vi "Get Default Name From TD.vi"(8 "错误输入":errorcluster, 10 "Type Descriptor":T1) -> (0 "错误输出":errorcluster, 2 "Name":string)   [LabVIEW 2012, in "TD Tools.lvlib"]
uses:
  TD Tools.lvlib
  Custom Type/Type Descriptor.ctl
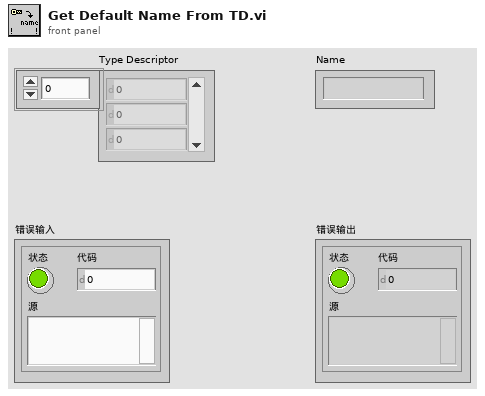
[diagram p1: front panel]
types:
  T1 = typedef "TD Tools.lvlib/Type Descriptor.ctl" = u16[]
  T2 = typedef "TD Tools.lvlib/Type Descriptor Header.ctl" = cluster{"length":u16, "private":u8, "type":T3, "# elements":u16}
  T3 = typedef "TD Tools.lvlib/Type Descriptor Enumeration.ctl" = enum16{"<Null>", "I8", "I16", "I32", "I64", "U8", "U16", "U32", "U64", "SGL", "DBL", "EXT", "CSG", "CDB", "CXT", "0x0F", "0x10", "0x11", "0x12", "0x13", "0x14", "Enum U8", "Enum U16", "Enum U32", "Enum U64", "SGL PQ", "DBL PQ", "EXT PQ", "CSG PQ", "CDB PQ", "CXT PQ", "0x1F", "0x20", "Boolean", "0x22", "0x23", "0x24", "0x25", "0x26", "0x27", "0x28", "0x29", "0x2A", "0x2B", "0x2C", "0x2D", "0x2E", "0x2F", "String", "0x31", "Path", "Pict", "0x34", "0x35", "0x36", "DAQ", "0x38", "0x39", "0x3A", "0x3B", "0x3C", "0x3D", "0x3E", "0x3F", "Array", "0x41", "0x42", "0x43", "0x44", "0x45", "0x46", "0x47", "0x48", "0x49", "0x4A", "0x4B", "0x4C", "0x4D", "0x4E", "0x4F", "Cluster", "0x51", "0x52", "Variant", "Waveform", "0x55", "0x56", "0x57", "0x58", "0x59", "0x5A", "0x5B", "0x5C", "0x5D", "0x5E", "0x5F", "0x60", "0x61", "0x62", "0x63", "0x64", "0x65", "0x66", "0x67", "0x68", "0x69", "0x6A", "0x6B", "0x6C", "0x6D", "0x6E", "0x6F", "Refnum"}
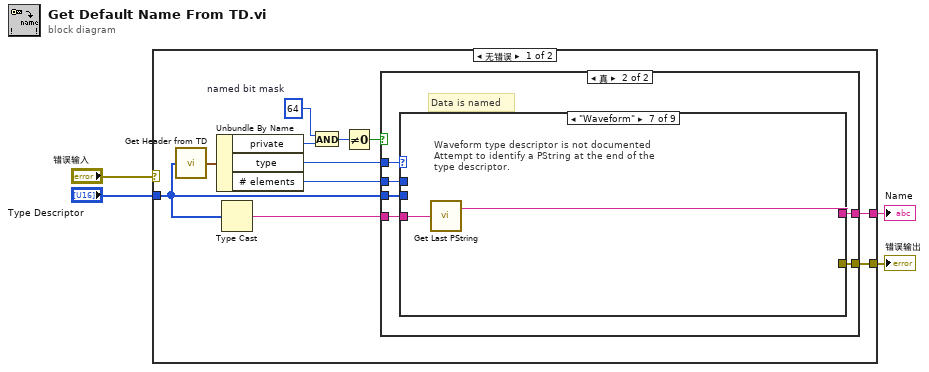
[diagram p0: block diagram]
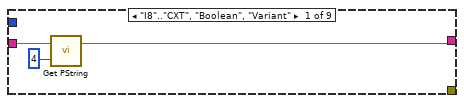
[diagram p3: hidden frame]
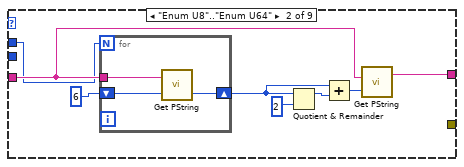
[diagram p4: hidden frame]
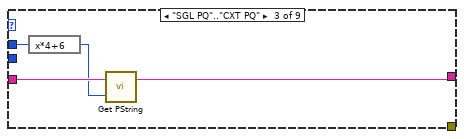
[diagram p5: hidden frame]
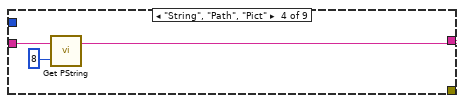
[diagram p6: hidden frame]
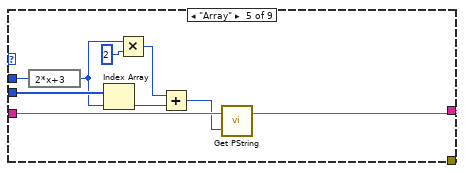
[diagram p7: hidden frame]
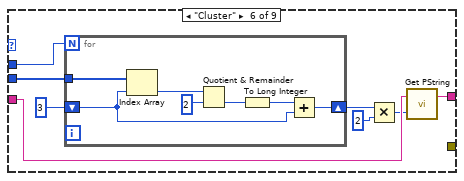
[diagram p8: hidden frame]
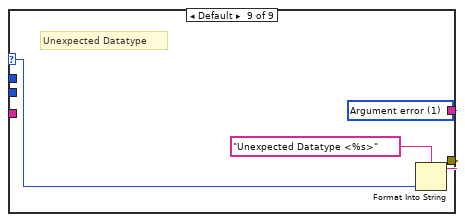
[diagram p10: hidden frame]
diagram:
  n1 = case shown="无错误" "错误输入" {
    selector: "错误输入" -> [_ w77]
    tunnel: "Type Descriptor" -> [w14 _]
    tunnel: [w11 "" ("Last PString")] -> w3
    tunnel: [w5 w77] -> w1
    frame No Error {
      w8 = u8 64  # named bit mask
      n2 = call "Get Header from TD.vi"("Type Desciptor"=w14) -> ("Type Descriptor Header"=w15:T2)
      n3 = Unbundle By Name(w15) -> ("private"=w7:u8, "type"=w6:T3, "# elements"=w13:u16)
      n4 = Type Cast(x=w14) -> (*(type *) &x=w12:string)  [unwired: 1 in]
      n5 = And(x=w8, y=w7) -> (x .and. y?=w10:u8)
      n6 = Not Equal To 0?(x=w10) -> (x != 0?=w9:bool)
      n7 = case shown="真" w9 {
        tunnel: [_ w21] -> w5
        tunnel: w6 -> [_ w20]
        tunnel: w12 -> [_ w19]
        tunnel: [_ w18] -> w11
        tunnel: w13 -> [_ w17]
        tunnel: w14 -> [_ w16]
        frame False {
        }
        frame True {
          # "Data is named"
          n8 = case shown="\"Waveform\"" w20 {
            selector: w20 -> [_ _ _ _ _ _ _ _ w71]
            tunnel: [_ _ _ _ _ _ _ _ w75] -> w21
            tunnel: w19 -> [w24 w29 w38 w42 w49 w57 w68 w70 _]
            tunnel: [w22 w28 w36 w41 w48 w56 w67 w69 _] -> w18
            tunnel: w17 -> [_ w27 w39 _ w51 w59 _ _ _]
            tunnel: w16 -> [_ _ _ _ w50 w58 _ _ _]
            frame "I8".."CXT", "Boolean", "Variant" {
              n9 = call "Get PString.vi"("offset(0)"=4 ("offset (0)"), "String"=w24) -> ("PString"=w22:string)  [unwired: 1 out]
            }
            frame "Enum U8".."Enum U64" {
              n10 = for {
                N: w27 -> [_]
                tunnel: w29 -> [w33]
                shift-right: [w34] -> w31
                shift-left: 6 -> [w35]
                n11 = call "Get PString.vi"("offset(0)"=w35, "String"=w33) -> ("offset  Past PString"=w34:i32)  [unwired: 1 out]
              }
              n12 = Quotient & Remainder(x=w31, y=2) -> (x-y*floor(x/y)=w25:i32)  [unwired: 1 out]
              n13 = Add(x=w31, y=w25) -> (x+y=w30:i32)
              n14 = call "Get PString.vi"("offset(0)"=w30, "String"=w29) -> ("PString"=w28:string)  [unwired: 1 out]
            }
            frame "SGL PQ".."CXT PQ" {
              n15 = expression code="x*4+6"(w39) -> (w37:u16)
              n16 = call "Get PString.vi"("offset(0)"=w37, "String"=w38) -> ("PString"=w36:string)  [unwired: 1 out]
            }
            frame "String", "Path", "Pict" {
              n17 = call "Get PString.vi"("offset(0)"=8 ("offset (0)"), "String"=w42) -> ("PString"=w41:string)  [unwired: 1 out]
            }
            frame "Array" {
              n18 = expression code="2*x+3"(w51) -> (w47:u16)
              n19 = Index Array(array=w50, index=w47) -> (element=w44:u16)
              n20 = Multiply(x=w47, y=u16 2) -> (x*y=w45:u16)
              n21 = Add(x=w45, y=w44) -> (x+y=w43:u16)
              n22 = call "Get PString.vi"("offset(0)"=w43, "String"=w49) -> ("PString"=w48:string)  [unwired: 1 out]
            }
            frame "Cluster" {
              n23 = for {
                N: w59 -> [_]
                shift-right: [w65] -> w54
                shift-left: 3 -> [w64]
                tunnel: w58 -> [w66]
                n24 = Index Array(array=w66, index=w64) -> (element=w62:u16)
                n25 = Quotient & Remainder(x=w62, y=i16 2) -> (floor(x/y)=w63:u16)  [unwired: 1 out]
                n26 = To Long Integer(number=w63) -> (32bit integer=w60:i32)
                n27 = Add(x=w60, y=w64) -> (x+y=w65:i32)
              }
              n28 = Multiply(x=w54, y=2) -> (x*y=w53:i32)
              n29 = call "Get PString.vi"("offset(0)"=w53, "String"=w57) -> ("PString"=w56:string)  [unwired: 1 out]
            }
            frame "Waveform" {
              # "Waveform type descriptor is not documented\nAttempt to identify a PString at the end of the\ntype descriptor."
              n30 = call "Get Last PString.vi"("String"=w68) -> ("Last String"=w67:string)  [unwired: 1 out]
            }
            frame "DAQ", "Refnum" {
              # "Refnums type descriptors are not documented\nAttempt to identify a PString at the end of the\ntype descriptor."
              n31 = call "Get Last PString.vi"("String"=w70) -> ("Last String"=w69:string)  [unwired: 1 out]
            }
            frame Default {
              w74 = 1 items=["No error", "Argument error", "Memory is full", "Out of zone", "End of file", "File already open", "Generic file I/O error", "File not found", "File permission error", "Disk is full", "Duplicate path", "Too many files open", "System feature not enabled", "Resource file not found", "Cannot add resource", "Resource not found", "Image not found", "Image memory error", "Pen does not exist", "Config type invalid", "Config token not found", "Config parse error", "Config memory error", "Bad external code format", "Bad external code offset", "External code not present", "Null window", "Destroy window error", "Null menu", "Print aborted", "Bad print record", "Print driver error", "Windows error during printing", "Memory error during printing", "Print dialog error", "Generic print error", "Invalid device refnum", "Device not found", "Device parameter error", "Device unit error", "Cannot open device", "Device call aborted", "Generic error", "Cancelled by user", "Object ID too low", "Object ID too high", "Object not in heap", "Unknown heap", "Unknown object (invalid DefProc)", "Unknown object (DefProc not in table)", "Message out of range", "Invalid (null) method", "Unknown message", "Manager call not supported", "Bad address", "Network operation in progress", "Network operation timed out", "Connection is busy", "Network attribute not supported", "Network error", "Address in use", "System out of memory", "Connection aborted", "Connection refused", "Not connected", "Already connected", "Connection closed", "Initialization error (interapplication manager)", "Bad occurrence", "Wait on unbound occurrence handler", "Occurrence queue overflow", "Datalog type conflict", "Unused", "Unrecognized type (interapplication manager)", "Memory corrupt", "Failed to make temporary DLL", "Old CIN version", "Drag socket not found", "Failed to load drop-object", "Failed to register OLE object", "Failed to release OLE object", "Format specifier type mismatch", "Unknown format specifier", "Too few format specifiers", "Too many format specifiers", "Scan failed", "Newer CIN version", "Error converting to variant", "Runtime menu error", "Password tampered", "Variant attribute not found", "Incompatible variant data type", "Event data is not available", "Event Store is not present", "Occurrence is not found", "Event Queue is not created", "Event info is not available", "Refnum passed is NULL", "Error retrieving Class GUID", "Error retrieving CoClass GUID", "Error retrieving TypeLib GUID.", "Bad built application magic bytes.", "Specific driver is different from the specific driver associated with the Logical Name.", "There is no session opened to the class driver.", "Max Error", "MAX - Error with config objects", "MAX - Error loading configuration", "MAX - Group not supported"]
              # "Unexpected Datatype"
              n32 = Format Into String(format string="Unexpected Datatype <%s>" ("Format String"), w71) -> (resulting string=w72:string)  [unwired: 2 in, 1 out]
              n33 = call "Build Error Cluster.vi"("String to Prepend to source (\"\")"=w72, "code"=w74) -> ("error out"=w75:errorcluster)
            }
          }
        }
      }
    }
    frame Error {
    }
  }
  "Name" <- w3
  "错误输出" <- w1
